vi "SinSignalMessage.vi"(6 "Offset":dbl, 7 "Filter":T1, 8 "Phase":dbl, 9 "Amplitude":dbl, 10 "Frequency":dbl, 11 "OutputStage":T2) -> (3 "SineSignalMessage":string)   [LabVIEW 2016]
uses:
  OutputStageTypeDef.ctl
  FilterTypeDef.ctl
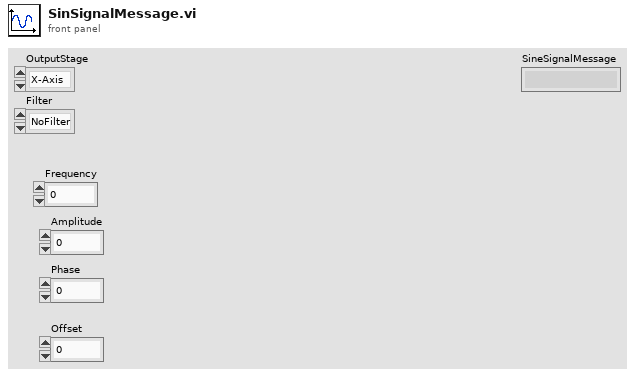
[diagram p1: front panel]
types:
  T1 = typedef "FilterTypeDef.ctl" = enum16{"NoFilter", "Bessel6thOrder300"}
  T2 = typedef "OutputStageTypeDef.ctl" = enum16{"X-Axis", "Y-Axis"}
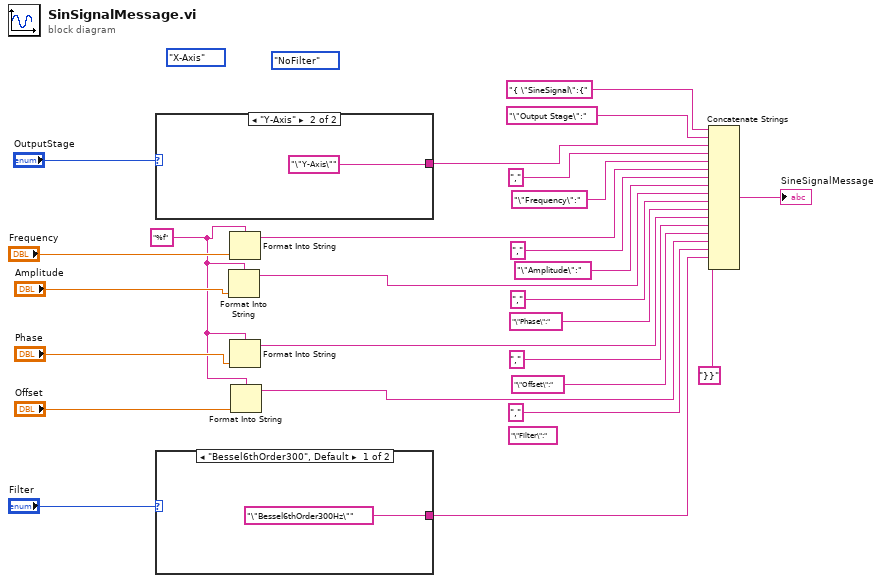
[diagram p0: block diagram]
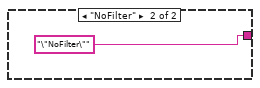
[diagram p2: hidden frame]
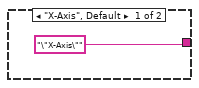
[diagram p3: hidden frame]
diagram:
  (unwired) "\"Filter\":"
  w1 = "%f" ("initial string")
  (unwired) FilterTypeDef."NoFilter"
  (unwired) OutputStageTypeDef."X-Axis"
  n1 = case shown="\"Y-Axis\"" "OutputStage" {
    tunnel: ["\"X-Axis\"" "\"Y-Axis\""] -> w22
    frame "X-Axis", Default {
    }
    frame "Y-Axis" {
    }
  }
  n2 = case shown="\"Bessel6thOrder300\", Default" "Filter" {
    tunnel: ["\"Bessel6thOrder300Hz\"" "\"NoFilter\""] -> w4
    frame "Bessel6thOrder300", Default {
    }
    frame "NoFilter" {
    }
  }
  n3 = Format Into String(format string=w1, "Amplitude") -> (resulting string=w12:string)  [unwired: 2 in, 1 out]
  n4 = Format Into String(format string=w1, "Frequency") -> (resulting string=w15:string)  [unwired: 2 in, 1 out]
  n5 = Format Into String(format string=w1, "Phase") -> (resulting string=w9:string)  [unwired: 2 in, 1 out]
  n6 = Format Into String(format string=w1, "Offset") -> (resulting string=w6:string)  [unwired: 2 in, 1 out]
  n7 = Concatenate Strings("{ \"SineSignal\":{", "\"Output Stage\":", w22, ",", "\"Frequency\":", w15, ",", "\"Amplitude\":", w12, ",", "\"Phase\":", w9, ",", "\"Offset\":", w6, ",", w4, "}}" ("string")) -> (→"SineSignalMessage":string)
